vi "Spectral Measurements.vi"() -> ()   [LabVIEW 2023]
uses:
  <vilib>/express/express analysis/Spectral/Block/exnSpectralBlock spectral measurements PSD poly.vi
  <vilib>/express/express analysis/Spectral/Block/exnSpectralBlock spectral measurements PSD DDT.vi
  <vilib>/express/express analysis/Spectral/XNode/ExpressSpectralMeasurementsBlockNode.xnode
panel:
  in  "?":bool
  in  "Frequency(Hz)":dbl(slide) scale=0.0..100.0
  out "Waveform Graph":dynamicdata(graph)
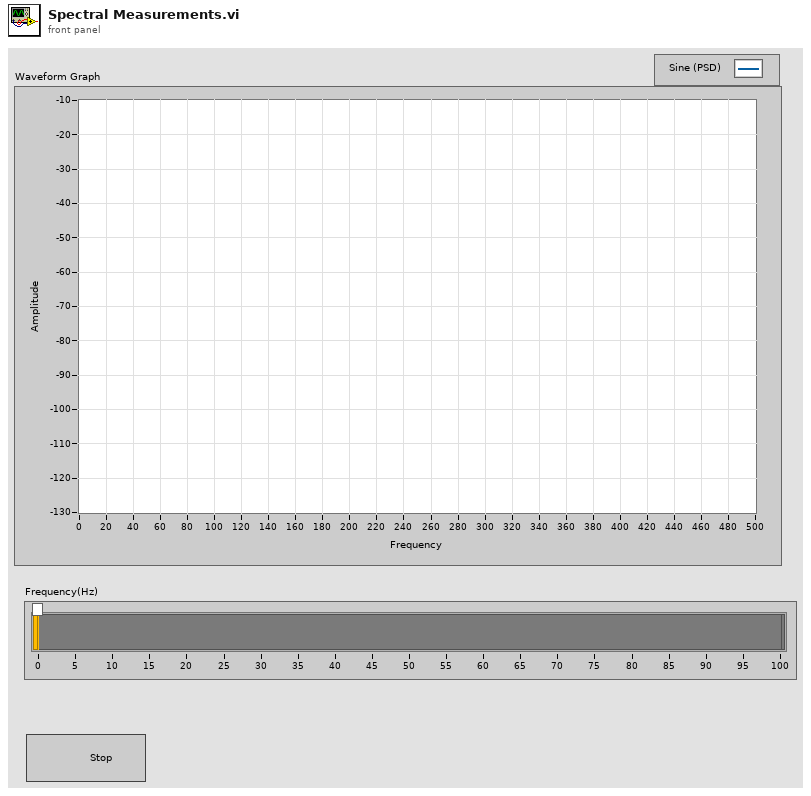
[diagram p1: front panel]
types:
  T1 = cluster{"averaging mode":u16, "weighting mode":u16, "number of averages":u32}
  T2 = cluster{"dB On (F)":bool, "unwrap phase (F)":bool, "convert to degree (F)":bool}
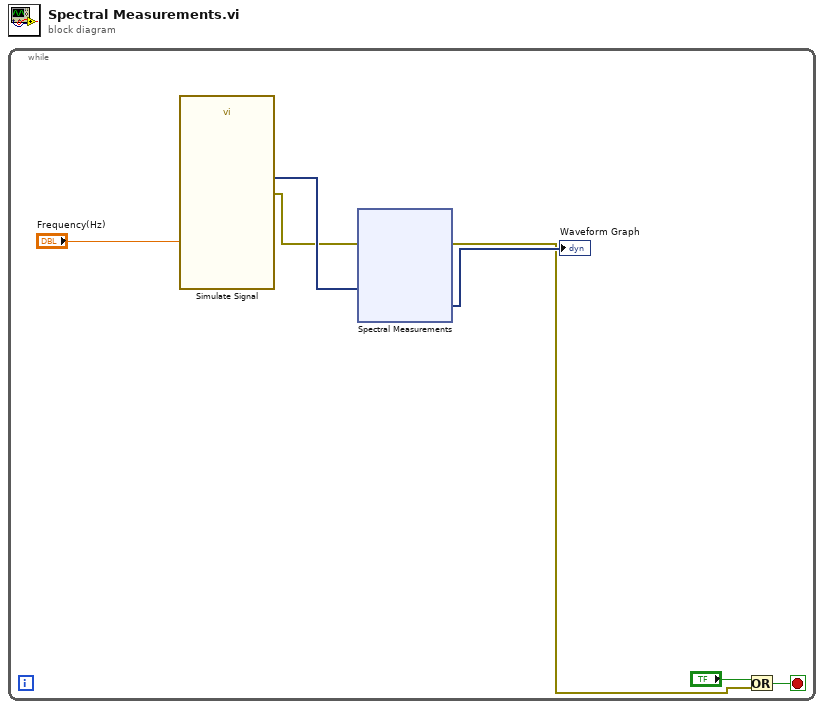
[diagram p0: block diagram]
diagram:
  n1 = while {
    stop <- w6 stop-if-true
    n2 = call "Simulate Signal"("Frequency"="Frequency(Hz)") -> ("Sine"=w3:dynamicdata, "error out"=w2:errorcluster)  [unwired: 13 in]
    n3 = xnode "Spectral Measurements"("Signals"=w3, "error in (no error)"=w2) -> ("PSD"=→"Waveform Graph":dynamicdata, "error out"=w1:errorcluster)
    n4 = Or(x="?", y=w1) -> (x .or. y?=w6:bool)
  }
